vi "InputText.vi"(11 "Caption.Text":string) -> (3 "ok?":bool)   [LabVIEW 2016]
uses:
  InfoGui.Action.ctl
  tools/Config/Config.Global.vi
panel:
  out "_loop":i32(ring)=4
  in  "InputText":string
  in  "CancelButton":bool
  in  "OKButton":bool
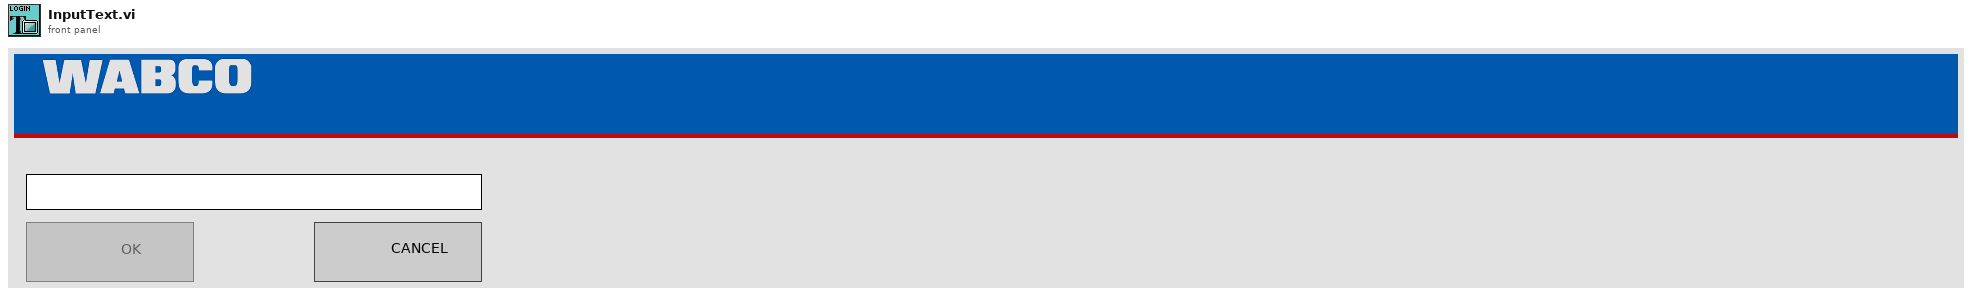
[diagram p1: front panel]
types:
  T1 = typedef "InfoGui.Action.ctl" = enum32{"idle", "constructor", "destructor", "--- InfoGUI ---"}
  T2 = enum8{"Enabled", "Disabled", "Disabled and Grayed Out"}
  T3 = enum32{"Invalid", "Default", "Floating", "Floating/Auto-Hide", "Modal"}
  T4 = typedef "FestoCPX.Station.ButtonsState.ctl" = cluster{"Start":bool, "Stop":bool, "Control":bool}
  T5 = typedef "LVPositionTypeDef.ctl" = cluster{"Left":i32, "Top":i32}
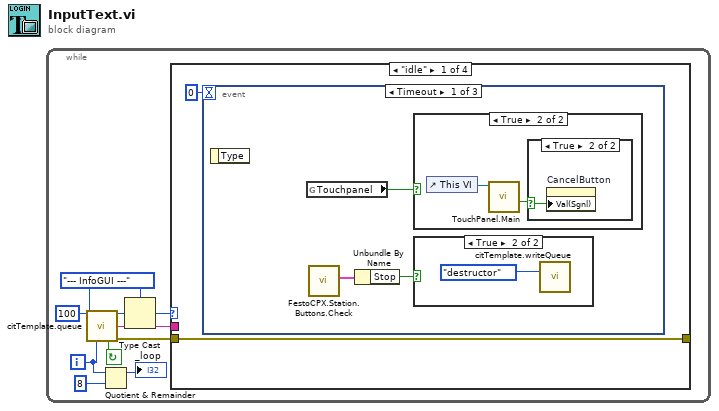
[diagram p0: block diagram]
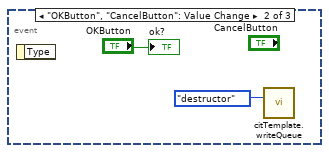
[diagram p5: hidden frame]
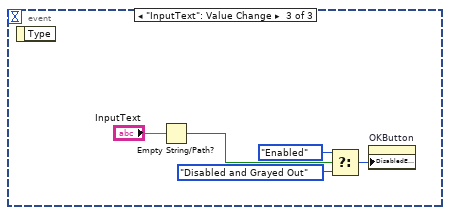
[diagram p6: hidden frame]
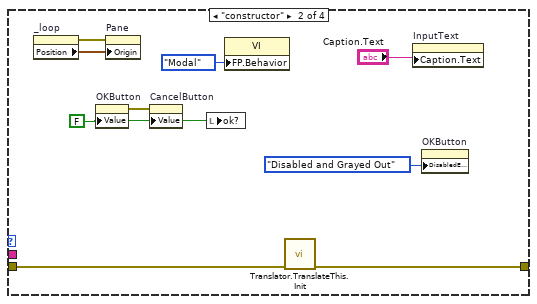
[diagram p7: hidden frame]
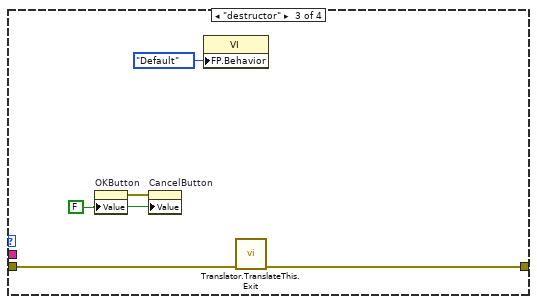
[diagram p8: hidden frame]
diagram:
  n1 = while {
    i -> [w1]
    stop <- w7 continue-if-true
    w6 = InfoGui.Action."--- InfoGUI ---" ("Action")
    n2 = call "citTemplate.queue.vi"("ms timeout (250 ms)"=100, "event enum"=w6, "iteration (-1)"=w1) -> ("event out"=w10:u32, "(flatten) data out"=w9:string, "continue"=w7:bool, "error out"=w8:errorcluster)  [unwired: 2 in, 7 out]
    n3 = Quotient & Remainder(x=w1, y=8) -> (x-y*floor(x/y)=→"_loop":i32)  [unwired: 1 out]
    n4 = Type Cast(type=w6, x=w10) -> (*(type *) &x=w5:T1)
    n5 = case shown="\"idle\"" w5 {
      tunnel: w9 -> [_ _ _ _]
      tunnel: w8 -> [w11 w31 w38 w41]
      tunnel: [w11 w30 w37 w41] -> _
      frame "idle" {
        n6 = event shown="[0] Timeout" {
          selector: _ -> [_ _ _]
          dyn-events: _ -> [_ _ _]
          timeout: 0 -> [_ _ _]
          event Timeout {
            n7 = event-data() -> ()  [unwired: 1 in, 1 out]
            n8 = global read "Config.Global.vi" "Touchpanel"() -> (w15:bool)
            n9 = call "FestoCPX.Station.Buttons.Check.vi"() -> ("Buttons.State"=w14:T4)  [unwired: 10 in, 1 out]
            n10 = Unbundle By Name(w14) -> ("Stop"=w13:bool)
            n11 = case shown="True" w15 {
              frame False {
              }
              frame True {
                n12 = control-ref of="This VI"() -> (w18:refnum<vi>)
                n13 = call "TouchPanel.Main.vi"("VI ref"=w18) -> ("Canceled"=w17:bool)  [unwired: 8 in, 2 out]
                n14 = case shown="True" w17 {
                  selector: w17 -> [_ w19]
                  frame False {
                  }
                  frame True {
                    n15 = property on="CancelButton" class="Bool (strict)"("Val(Sgnl)"=w19) -> ()  [unwired: 2 in, 2 out]
                  }
                }
              }
            }
            n16 = case shown="True" w13 {
              frame False {
              }
              frame True {
                n17 = call "citTemplate.writeQueue.vi"("event in (if not connected:all statemachine with data event)"=InfoGui.Action."destructor" ("Action")) -> ()  [unwired: 14 in, 1 out]
              }
            }
          }
          event "OKButton", "CancelButton": Value Change {
            n18 = event-data() -> ()  [unwired: 1 in, 1 out]
            n19 = call "citTemplate.writeQueue.vi"("event in (if not connected:all statemachine with data event)"=InfoGui.Action."destructor" ("Action")) -> ()  [unwired: 14 in, 1 out]
            "ok?" <- "OKButton"
          }
          event "InputText": Value Change {
            n20 = event-data() -> ()  [unwired: 1 in, 1 out]
            n21 = Empty String/Path?(string/path="InputText") -> (empty?=w22:bool)
            n22 = Select(t=T2."Enabled" ("Disabled"), s=w22, f=T2."Disabled and Grayed Out" ("Disabled")) -> (s? t:f=w25:T2)
            n23 = property on="OKButton" class="Bool (strict)"("DisabledEnum"=w25) -> ()  [unwired: 2 in, 2 out]
          }
        }
      }
      frame "constructor" {
        w34 = FALSE ("_b_OK")
        n24 = property on="_loop" class="Ring (strict)"() -> (error out=w32:errorcluster, "Position"=w33:T5)  [unwired: 2 in, 1 out]
        n25 = property on="OKButton" class="Bool (strict)"("Value"=w34) -> (error out=w35:errorcluster)  [unwired: 2 in, 1 out]
        n26 = property on="Pane" class="Pane"(error in=w32, "Origin"=w33) -> ()  [unwired: 1 in, 2 out]
        n27 = property on="CancelButton" class="Bool (strict)"(error in=w35, "Value"=w34) -> ()  [unwired: 1 in, 2 out]
        n28 = local write "ok?"(w34) -> ()
        n29 = property class="VI"("FP.Behavior"=T3."Modal" ("Front Panel Window:Behavior")) -> ()  [unwired: 2 in, 2 out]
        n30 = call "Translator.TranslateThis.Init.vi"("error in"=w31) -> ("error out"=w30:errorcluster)  [unwired: 10 in]
        n31 = property on="InputText" class="Str"("Caption.Text"="Caption.Text") -> ()  [unwired: 2 in, 2 out]
        n32 = property on="OKButton" class="Bool (strict)"("DisabledEnum"=T2."Disabled and Grayed Out" ("Disabled")) -> ()  [unwired: 2 in, 2 out]
      }
      frame "destructor" {
        w39 = FALSE ("_b_OK")
        n33 = property on="OKButton" class="Bool (strict)"("Value"=w39) -> (error out=w40:errorcluster)  [unwired: 2 in, 1 out]
        n34 = property on="CancelButton" class="Bool (strict)"(error in=w40, "Value"=w39) -> ()  [unwired: 1 in, 2 out]
        n35 = property class="VI"("FP.Behavior"=T3."Default" ("Front Panel Window:Behavior")) -> ()  [unwired: 2 in, 2 out]
        n36 = call "Translator.TranslateThis.Exit.vi"("error in"=w38) -> ("error out"=w37:errorcluster)  [unwired: 10 in]
      }
      frame "--- InfoGUI ---" {
      }
    }
  }
